vi "Send HTML Email.vi"(8 "error in (no error)":errorcluster, 10 "Second Batch":string[](array[string])=["Peng", "Wilbur", "Hafiz", "James"], 11 "First Batch":string[](array[string])=["Xue Sheng", "Denny", "Habib"]) -> (0 "error out":errorcluster, 2 "invalid recipients":string[](array[string]))   [LabVIEW 2016]
uses:
  <vilib>/smtpClient/Set Message Text Html.vi
  <vilib>/smtpClient/LabVIEWSMTPClient.lvlib
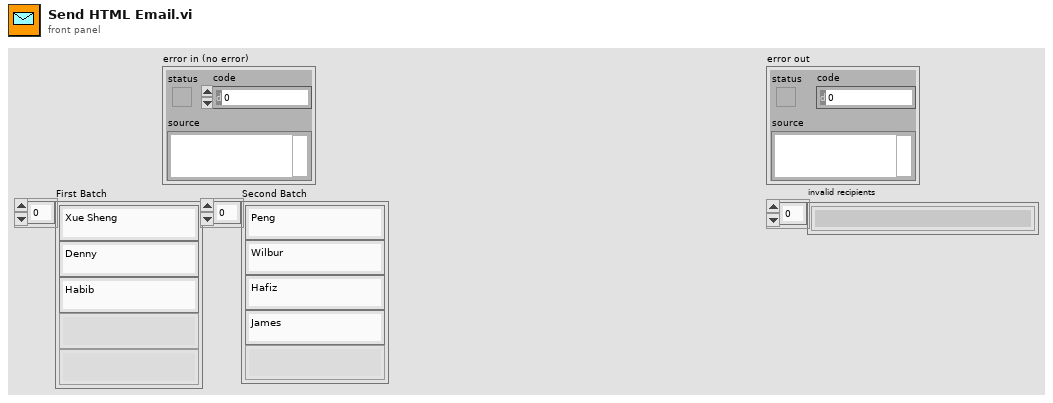
[diagram p1: front panel]
types:
  T1 = typedef "LabVIEWSMTPClient.lvlib/SmtpClientHandle.ctl" = refnum<k1>
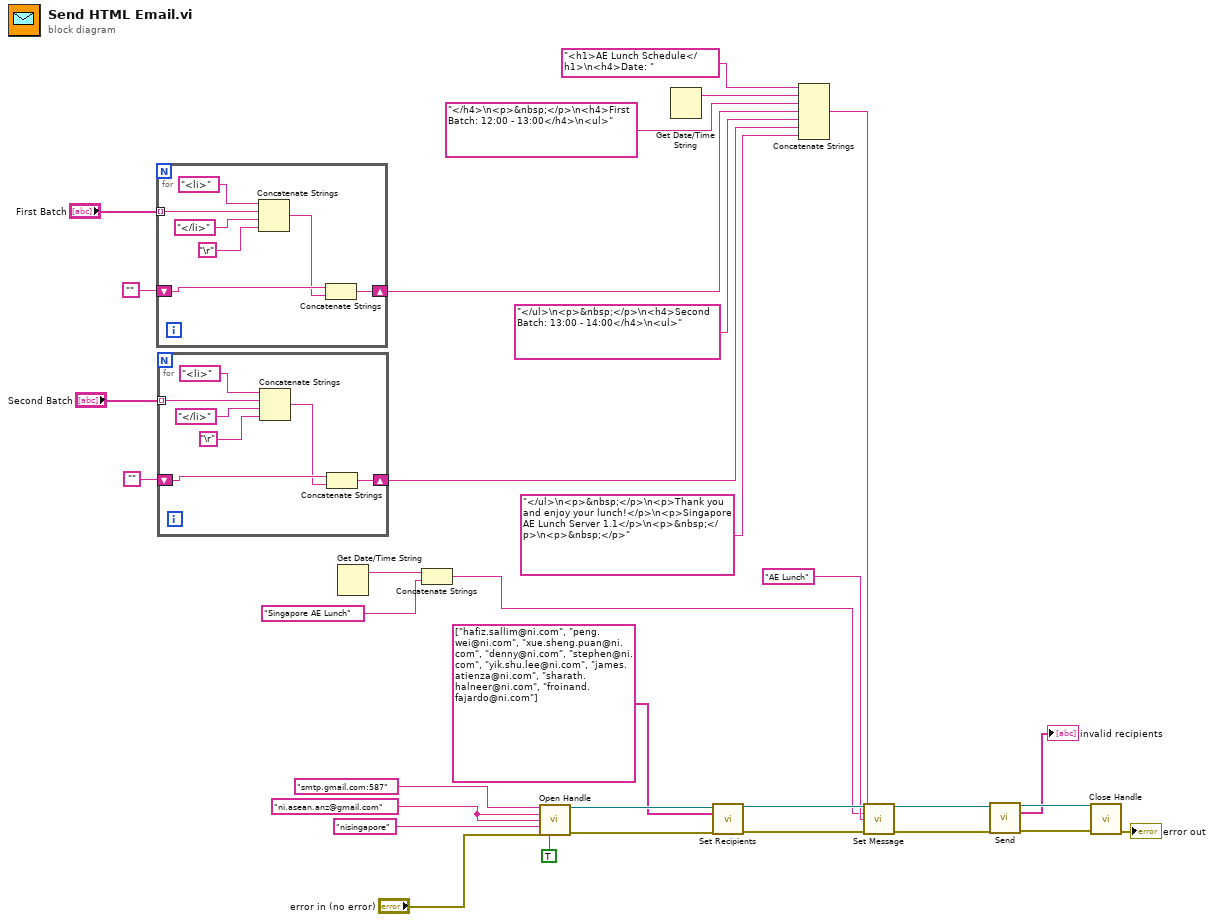
[diagram p0: block diagram]
diagram:
  w16 = "ni.asean.anz@gmail.com" ("from")
  n1 = for {
    tunnel: "First Batch" -> [w39] mode=indexing
    shift-right: [w33] -> w5
    shift-left: "" -> [w35]
    n2 = Concatenate Strings("<li>", w39, "</li>", "\r") -> (w34:string)
    n3 = Concatenate Strings(w35, w34) -> (w33:string)
  }
  n4 = for {
    tunnel: "Second Batch" -> [w46] mode=indexing
    shift-right: [w40] -> w3
    shift-left: "" -> [w42]
    n5 = Concatenate Strings("<li>", w46, "</li>", "\r") -> (w41:string)
    n6 = Concatenate Strings(w42, w41) -> (w40:string)
  }
  n7 = Get Date/Time String() -> (date string=w15:string)  [unwired: 3 in, 1 out]
  n8 = Concatenate Strings(w15, "Singapore AE Lunch" ("subject")) -> (w13:string)
  n9 = call <vilib>:"Open Handle.vi"("server address"="smtp.gmail.com:587", "from"=w16, "username"=w16, "password"="nisingapore", "error in (no error)"="error in (no error)", "use TLS (false)"=TRUE) -> ("handle out"=w31:T1, "error out"=w30:errorcluster)  [unwired: 8 in]
  n10 = Get Date/Time String() -> (date string=w7:string)  [unwired: 3 in, 1 out]
  n11 = call <vilib>:"Set Recipients.vi"("handle in"=w31, "to"=string[] ["hafiz.sallim@ni.com", "peng.wei@ni.com", "xue.sheng.puan@ni.com", "denny@ni.com", "stephen@ni.com", "yik.shu.lee@ni.com", "james.atienza@ni.com", "sharath.halneer@ni.com", "froinand.fajardo@ni.com"], "error in (no error)"=w30) -> ("handle out"=w28:T1, "error out"=w27:errorcluster)  [unwired: 11 in]
  n12 = Concatenate Strings("<h1>AE Lunch Schedule</h1>\n<h4>Date: ", w7, "</h4>\n<p>&nbsp;</p>\n<h4>First Batch: 12:00 - 13:00</h4>\n<ul>", w5, "</ul>\n<p>&nbsp;</p>\n<h4>Second Batch: 13:00 - 14:00</h4>\n<ul>", w3, "</ul>\n<p>&nbsp;</p>\n<p>Thank you and enjoy your lunch!</p>\n<p>Singapore AE Lunch Server 1.1</p>\n<p>&nbsp;</p>\n<p>&nbsp;</p>") -> (w1:string)
  n13 = call-poly <vilib>:"Set Message.vi"("handle in"=w28, "subject"=w13, "plain text message"="AE Lunch", "html message"=w1, "error in (no error)"=w27) -> ("handle out"=w24:T1, "error out"=w22:errorcluster)  [unwired: 9 in]
  n14 = call <vilib>:"Send.vi"("handle in"=w24, "error in (no error)"=w22) -> ("handle out"=w23:T1, "invalid recipients"=→"invalid recipients":string[], "error out"=w21:errorcluster)  [unwired: 11 in]
  n15 = call <vilib>:"Close Handle.vi"("handle in"=w23, "error in (no error)"=w21) -> ("error out"=→"error out":errorcluster)  [unwired: 12 in, 1 out]
